vi "CalcDistCluster.vi"(8 "Less than":dbl, 9 "element 2":cluster{"X":dbl, "Y":dbl, "Z":dbl}, 10 "element":cluster{"X":dbl, "Y":dbl, "Z":dbl}) -> (0 "Less than?":bool, 2 "Distance":dbl)   [LabVIEW 2014]
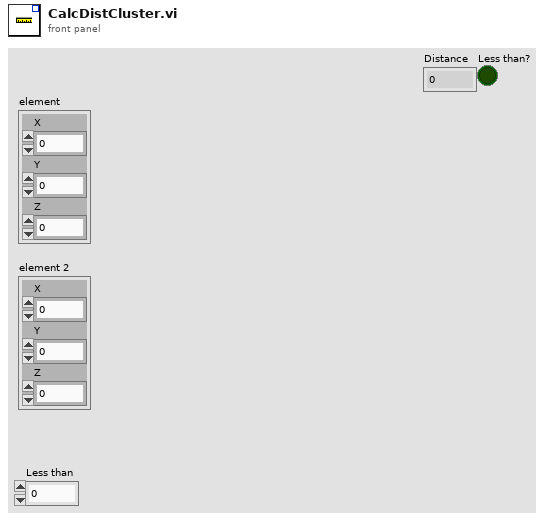
[diagram p1: front panel]
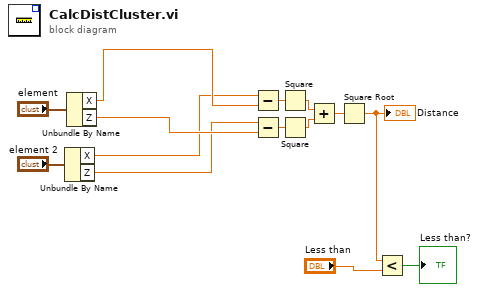
[diagram p0: block diagram]
diagram:
  n1 = Unbundle By Name("element 2") -> ("X"=w5:dbl, "Z"=w4:dbl)
  n2 = Unbundle By Name("element") -> ("X"=w7:dbl, "Z"=w6:dbl)
  n3 = Subtract(x=w5, y=w7) -> (x-y=w14:dbl)
  n4 = Subtract(x=w4, y=w6) -> (x-y=w13:dbl)
  n5 = Square(x=w14) -> (x^2=w11:dbl)
  n6 = Square(x=w13) -> (x^2=w12:dbl)
  n7 = Add(x=w11, y=w12) -> (x+y=w10:dbl)
  n8 = Square Root(x=w10) -> (sqrt(x)=w3:dbl)
  "Distance" <- w3
  n9 = Less?(x=w3, y="Less than") -> (x < y?=→"Less than?":bool)
